vi "Calculate Compression Ratio (SubVI).vi"(10 "N Compressed Packets":u32, 11 "Image Size":T1 {"Width" step=8; "Height" step=8}) -> (3 "Compression Ratio":dbl)   [LabVIEW 2015]
uses:
  Controls (HOST)/Image Size.ctl
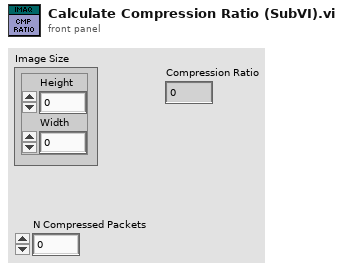
[diagram p1: front panel]
types:
  T1 = typedef "Image Size.ctl" = cluster{"Height":u16, "Width":u16}
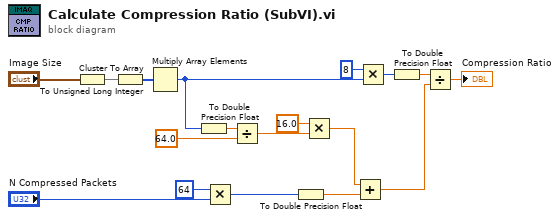
[diagram p0: block diagram]
diagram:
  n1 = Cluster To Array(cluster="Image Size") -> (array=w15:u16[])
  n2 = To Unsigned Long Integer(number=w15) -> (unsigned 32bit integer=w16:u32[])
  n3 = Multiply Array Elements(1:w16) -> (0:w6:u32)
  n4 = To Double Precision Float(number=w6) -> (double precision float=w7:dbl)
  n5 = Multiply(x=u32 64, y="N Compressed Packets") -> (x*y=w9:u32)
  n6 = Divide(x=w7, y=64.0) -> (x/y=w3:dbl)
  n7 = To Double Precision Float(number=w9) -> (double precision float=w10:dbl)
  n8 = Multiply(x=16.0, y=w3) -> (x*y=w1:dbl)
  n9 = Add(x=w1, y=w10) -> (x+y=w2:dbl)
  n10 = Multiply(x=u32 8, y=w6) -> (x*y=w13:u32)
  n11 = To Double Precision Float(number=w13) -> (double precision float=w11:dbl)
  n12 = Divide(x=w11, y=w2) -> (x/y=→"Compression Ratio":dbl)
